vi "Team Name to GID.vi"(10 "Teams in":T1(array[cluster]), 11 "Team Name":string) -> (3 "Team gid":string)   [LabVIEW 2016, in "Asana.lvclass"]
uses:
  levylab_expt_transport/src/Control Experiment/subVIs/Asana/Asana.lvclass
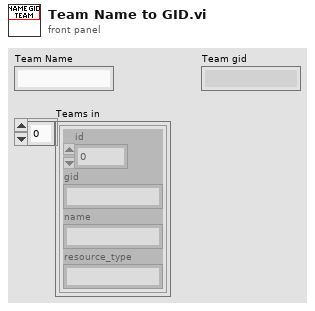
[diagram p1: front panel]
types:
  T1 = cluster{"id":i32, "gid":string, "name":string, "resource_type":string}[]
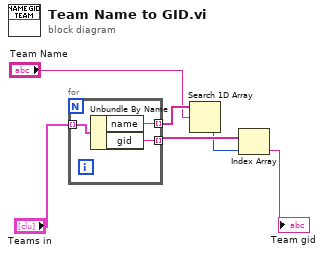
[diagram p0: block diagram]
diagram:
  n1 = for {
    tunnel: "Teams in" -> [w9] mode=indexing
    tunnel: [w8] -> w4 mode=indexing
    tunnel: [w7] -> w2 mode=indexing
    n2 = Unbundle By Name(w9) -> ("name"=w8:string, "gid"=w7:string)
  }
  n3 = Search 1D Array(1D array=w4, element="Team Name") -> (index of element=w1:i32)  [unwired: 1 in]
  n4 = Index Array(array=w2, index=w1) -> (element=→"Team gid":string)
